vi "TrajectoryExecuteAbsolute.vi"(8 "Init":bool, 11 "End Pose ENG":T1={"TRANSLATION"={"X"=0.0, "Y"=0.0}, "ROTATION"={"VALUE"=0.0, "COS"=1.0, "SIN"=0.0}} {"ROTATION"."SIN" format="%13.4f"; "ROTATION"."COS" format="%13.4f"; "ROTATION"."VALUE" format="%13.4f"; "TRANSLATION"."Y" format="%14.3f"; "TRANSLATION"."X" format="%14.3f"}) -> (0 "AtReference":bool, 3 "Chassis Velocity Target":T4 {"vOmega" format="%10.3f"; "vY" format="%10.3f"; "vX" format="%10.3f"})   [LabVIEW 2023]
uses:
  <vilib>/Rock Robotics/WPI/ThirdParty/JAS_Junk/TrajLib/TypeDef/CHASSIS_SPEEDS.ctl
  <vilib>/Rock Robotics/WPI/ThirdParty/JAS_Junk/TrajLib/TypeDef/POSE2D.ctl
  <vilib>/Rock Robotics/WPI/ThirdParty/JAS_Junk/TrajLib/TypeDef/TRANSLATION2D.ctl
  <vilib>/Rock Robotics/WPI/ThirdParty/JAS_Junk/TrajLib/TypeDef/ROTATION2D.ctl
  <vilib>/Rock Robotics/WPI/ThirdParty/JAS_Junk/TrajLib/VI/Util_GetTime_U32.vi
  <vilib>/Rock Robotics/WPI/ThirdParty/JAS_Junk/TrajLib/HolDrvCtrl_New.vi
  <vilib>/Rock Robotics/WPI/ThirdParty/JAS_Junk/TrajLib/HolDrvCtrl_PackPID.vi
  <vilib>/Rock Robotics/WPI/ThirdParty/JAS_Junk/TrajLib/HolDrvCtrl_SetTolerance.vi
  <vilib>/Rock Robotics/WPI/ThirdParty/JAS_Junk/TrajLib/HolDrvCtrl_SetEnabled.vi
  <vilib>/Rock Robotics/WPI/ThirdParty/JAS_Junk/TrajLib/HolDrvCtrl_Calculate_Trajectory.vi
  <vilib>/Rock Robotics/WPI/ThirdParty/JAS_Junk/TrajLib/HolDrvCtrl_AtReference.vi
  <vilib>/Rock Robotics/WPI/ThirdParty/JAS_Junk/TrajLib/ProfiledPIDController_NewPeriod.vi
  <vilib>/Rock Robotics/WPI/ThirdParty/JAS_Junk/TrajLib/ProfiledPIDController_SetIntegratorRange.vi
  <vilib>/Rock Robotics/WPI/ThirdParty/JAS_Junk/TrajLib/ProfiledPIDController_DisableContInput.vi
  <vilib>/Rock Robotics/WPI/ThirdParty/JAS_Junk/TrajLib/ProfiledPIDController_EnableContInput.vi
  <vilib>/Rock Robotics/WPI/ThirdParty/JAS_Junk/TrajLib/TrapProfConstraint_New.vi
  <vilib>/Rock Robotics/WPI/ThirdParty/JAS_Junk/TrajLib/Rotation2d_CreateAngle.vi
  <vilib>/Rock Robotics/WPI/ThirdParty/JAS_Junk/TrajLib/Translation2d_Create.vi
  <vilib>/Rock Robotics/WPI/ThirdParty/JAS_Junk/TrajLib/Conv_Deg_Radians.vi
  <vilib>/Rock Robotics/WPI/ThirdParty/JAS_Junk/TrajLib/PIDController_NewPeriod.vi
  <vilib>/Rock Robotics/WPI/ThirdParty/JAS_Junk/TrajLib/PIDController_SetIntegratorRange.vi
  <vilib>/Rock Robotics/WPI/ThirdParty/JAS_Junk/TrajLib/PIDController_Reset.vi
  <vilib>/Rock Robotics/WPI/ThirdParty/JAS_Junk/TrajLib/HolDrvCtrl_Calculate.vi
  <vilib>/Rock Robotics/WPI/ThirdParty/JAS_Junk/TrajLib/Rotation2d_GetRadians.vi
  <vilib>/Rock Robotics/WPI/ThirdParty/JAS_Junk/TrajLib/TrapProfState_New.vi
  <vilib>/Rock Robotics/SystemInterfaces/NetworkCommunication/NetComm_UsageReport_report.vi
  <vilib>/Rock Robotics/WPI/ThirdParty/JAS_Junk/TrajLib/PIDController_DisableContinousInput.vi
  <vilib>/Rock Robotics/WPI/ThirdParty/JAS_Junk/TrajLib/PIDController_EnableContinousInput.vi
  <vilib>/Rock Robotics/WPI/ThirdParty/JAS_Junk/TrajLib/Rotation2d_GetAngleCosSin.vi
  <vilib>/Rock Robotics/WPI/ThirdParty/JAS_Junk/TrajLib/Pose2d_RelativeTo.vi
  <vilib>/Rock Robotics/WPI/ThirdParty/JAS_Junk/TrajLib/Pose2d_getRotation.vi
  <vilib>/Rock Robotics/WPI/ThirdParty/JAS_Junk/TrajLib/Rotation2d_Minus.vi
  <vilib>/Rock Robotics/WPI/ThirdParty/JAS_Junk/TrajLib/ProfiledPIDController_Calculate_Meas_Goal.vi
  <vilib>/Rock Robotics/WPI/ThirdParty/JAS_Junk/TrajLib/PIDController_Calculate_SP_PV.vi
  <vilib>/Rock Robotics/WPI/ThirdParty/JAS_Junk/TrajLib/ProfiledPIDController_Reset_PosOnly.vi
  <vilib>/Rock Robotics/WPI/ThirdParty/JAS_Junk/TrajLib/ChassisSpeeds_FromFieldRelativeSpeeds.vi
  <vilib>/Rock Robotics/WPI/ThirdParty/JAS_Junk/TrajLib/Transform2d_Create_PosePose.vi
  <vilib>/Rock Robotics/WPI/ThirdParty/JAS_Junk/TrajLib/Pose2d_New_TRRO.vi
  <vilib>/Rock Robotics/WPI/ThirdParty/JAS_Junk/TrajLib/Rotation2d_UnaryMinus.vi
  <vilib>/Rock Robotics/WPI/ThirdParty/JAS_Junk/TrajLib/Rotation2d_RotateBy.vi
  <vilib>/Rock Robotics/WPI/ThirdParty/JAS_Junk/TrajLib/ProfiledPIDController_SetGoal_PosOnly.vi
  <vilib>/Rock Robotics/WPI/ThirdParty/JAS_Junk/TrajLib/ProfiledPIDController_Calculate_Meas.vi
  <vilib>/Rock Robotics/WPI/ThirdParty/JAS_Junk/TrajLib/PIDController_SetSetpoint.vi
  <vilib>/Rock Robotics/WPI/ThirdParty/JAS_Junk/TrajLib/PIDController_Calculate_PV.vi
  <vilib>/Rock Robotics/WPI/ThirdParty/JAS_Junk/TrajLib/ProfiledPIDController_Reset.vi
  <vilib>/Rock Robotics/WPI/ThirdParty/JAS_Junk/TrajLib/Rotation2d_GetCos.vi
  <vilib>/Rock Robotics/WPI/ThirdParty/JAS_Junk/TrajLib/Rotation2d_GetSin.vi
  <vilib>/Rock Robotics/WPI/ThirdParty/JAS_Junk/TrajLib/Translation2d_RotateBy.vi
  <vilib>/Rock Robotics/WPI/ThirdParty/JAS_Junk/TrajLib/Translation2d_Minus.vi
  <vilib>/Rock Robotics/WPI/ThirdParty/JAS_Junk/TrajLib/Rotation2d_CreateXY.vi
  <vilib>/Rock Robotics/WPI/ThirdParty/JAS_Junk/TrajLib/ProfiledPIDController_SetGoal.vi
  <vilib>/Rock Robotics/WPI/ThirdParty/JAS_Junk/TrajLib/TrapProfile_New.vi
  <vilib>/Rock Robotics/WPI/ThirdParty/JAS_Junk/TrajLib/ProfiledPIDController_GetPeriod.vi
  <vilib>/Rock Robotics/WPI/ThirdParty/JAS_Junk/TrajLib/TrapProfile_Calculate.vi
  <vilib>/Rock Robotics/WPI/ThirdParty/JAS_Junk/TrajLib/ControllerUtil_GetModulusError.vi
  <vilib>/Rock Robotics/WPI/ThirdParty/JAS_Junk/TrajLib/Util_CalcDist.vi
  <vilib>/Rock Robotics/WPI/ThirdParty/JAS_Junk/TrajLib/TrapProfile_ShouldFlipAcceleration.vi
  <vilib>/Rock Robotics/WPI/ThirdParty/JAS_Junk/TrajLib/TrapProfile_Direct.vi
  <vilib>/Rock Robotics/WPI/ThirdParty/JAS_Junk/TrajLib/PIDController_GetPeriod.vi
  Vision/VisionGlobal.vi
  TrajectoryGlobals.vi
  <vilib>/Rock Robotics/SystemInterfaces/Utilities/FPGA_UtilitiesRead LocalTime.vi
  <vilib>/Rock Robotics/WPI/ThirdParty/JAS_Junk/TrajLib/VI/Util_GetTime_U64.vi
  <vilib>/Rock Robotics/WPI/ThirdParty/JAS_Junk/TrajLib/Globals/Util_LibraryGlobals.vi
  <vilib>/Rock Robotics/WPI/ThirdParty/JAS_Junk/TrajLib/Trajectory_Library.lvlib
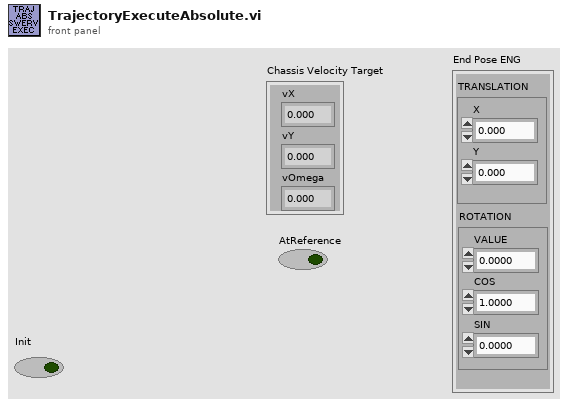
[diagram p1: front panel]
types:
  T1 = typedef "Trajectory_Library.lvlib/POSE2D.ctl" = cluster{"TRANSLATION":T2, "ROTATION":T3}
  T2 = typedef "Trajectory_Library.lvlib/TRANSLATION2D.ctl" = cluster{"X":dbl, "Y":dbl}
  T3 = typedef "Trajectory_Library.lvlib/ROTATION2D.ctl" = cluster{"VALUE":dbl, "COS":dbl, "SIN":dbl}
  T4 = typedef "Trajectory_Library.lvlib/CHASSIS_SPEEDS.ctl" = cluster{"vX":dbl, "vY":dbl, "vOmega":dbl}
  T5 = typedef "Trajectory_Library.lvlib/SWERVE_DRIVE_KINEMATICS.ctl" = cluster{"NumModules":i32, "InverseKinematics":T6, "ForwardKinematics":T6, "Modules":T2[], "PrevCoR":T2, "SavedModuleStates":T7[]}
  T6 = typedef "NI_Matrix.lvlib/RealMatrix.ctl" = dbl[][]
  T7 = typedef "Trajectory_Library.lvlib/SWERVE_DRIVE_MODULE_STATE.ctl" = cluster{"Speed":dbl, "Angle":T3}
  T8 = typedef "Trajectory_Library.lvlib/TRAJECTORY.ctl" = cluster{"TotalTImeSecs":dbl, "States":T9[]}
  T9 = typedef "Trajectory_Library.lvlib/TRAJ_STATE.ctl" = cluster{"TimeSeconds":dbl, "Velocity":dbl, "Acceleration":dbl, "POSE":T1, "Curvature":dbl}
  T10 = typedef "Trajectory_Library.lvlib/PID_TUNING.ctl" = cluster{"Kp":dbl, "Ki":dbl, "Kd":dbl, "MaximumIntegral":dbl, "MinimumIntegral":dbl, "IntegralZone":dbl}
  T11 = typedef "Trajectory_Library.lvlib/PROFILED_PID_CONTROLLER.ctl" = cluster{"Controller":T12, "Goal":T13, "Setpoint":T13, "Constraint":T14}
  T12 = typedef "Trajectory_Library.lvlib/PID_CONTROLLER.ctl" = cluster{"Kp":dbl, "Ki":dbl, "Kd":dbl, "Period":dbl, "Max_Integral":dbl, "Min_Integral":dbl, "Max_Input":dbl, "Min_Input":dbl, "Continuous":bool, "PositionError":dbl, "VelocityError":dbl, "PrevError":dbl, "Total_Integral":dbl, "PositionTolerance":dbl, "VelocityTolerance":dbl, "SetPoint":dbl, "Kf":dbl, "Prev_Deriv":dbl, "Prev_Deriv 2":dbl, "DerivativeFilter":bool, "Min_Output":dbl, "Max_Output":dbl, "Prev_F_P":dbl, "Prev_F_P_2":dbl, "AntiWindupActive":bool, "Measurement":dbl, "IntegralZone":dbl}
  T13 = typedef "Trajectory_Library.lvlib/TRAPEZOID_PROFILE_STATE.ctl" = cluster{"Position":dbl, "Velocity":dbl}
  T14 = typedef "Trajectory_Library.lvlib/TRAPEZOID_PROFILE_CONSTRAINT.ctl" = cluster{"MaxVelocity":dbl, "MaxAcceleration":dbl}
  T15 = typedef "Trajectory_Library.lvlib/HOLONOMIC_PACK_TUNING.ctl" = cluster{"X PID Tuning":T10, "Y PID Tuning":T10, "thetaProfiledPID_CTRL":T11}
  T16 = typedef "Trajectory_Library.lvlib/HOLONOMIC_DRV_CTRL.ctl" = cluster{"poseTolerance":T1, "poseError":T1, "Enabled":bool, "PID_xCtrl":T12, "PID_yCtrl":T12, "PROF_PID_thetaCtrl":T11, "RotationError":T3, "FirstRun":bool}
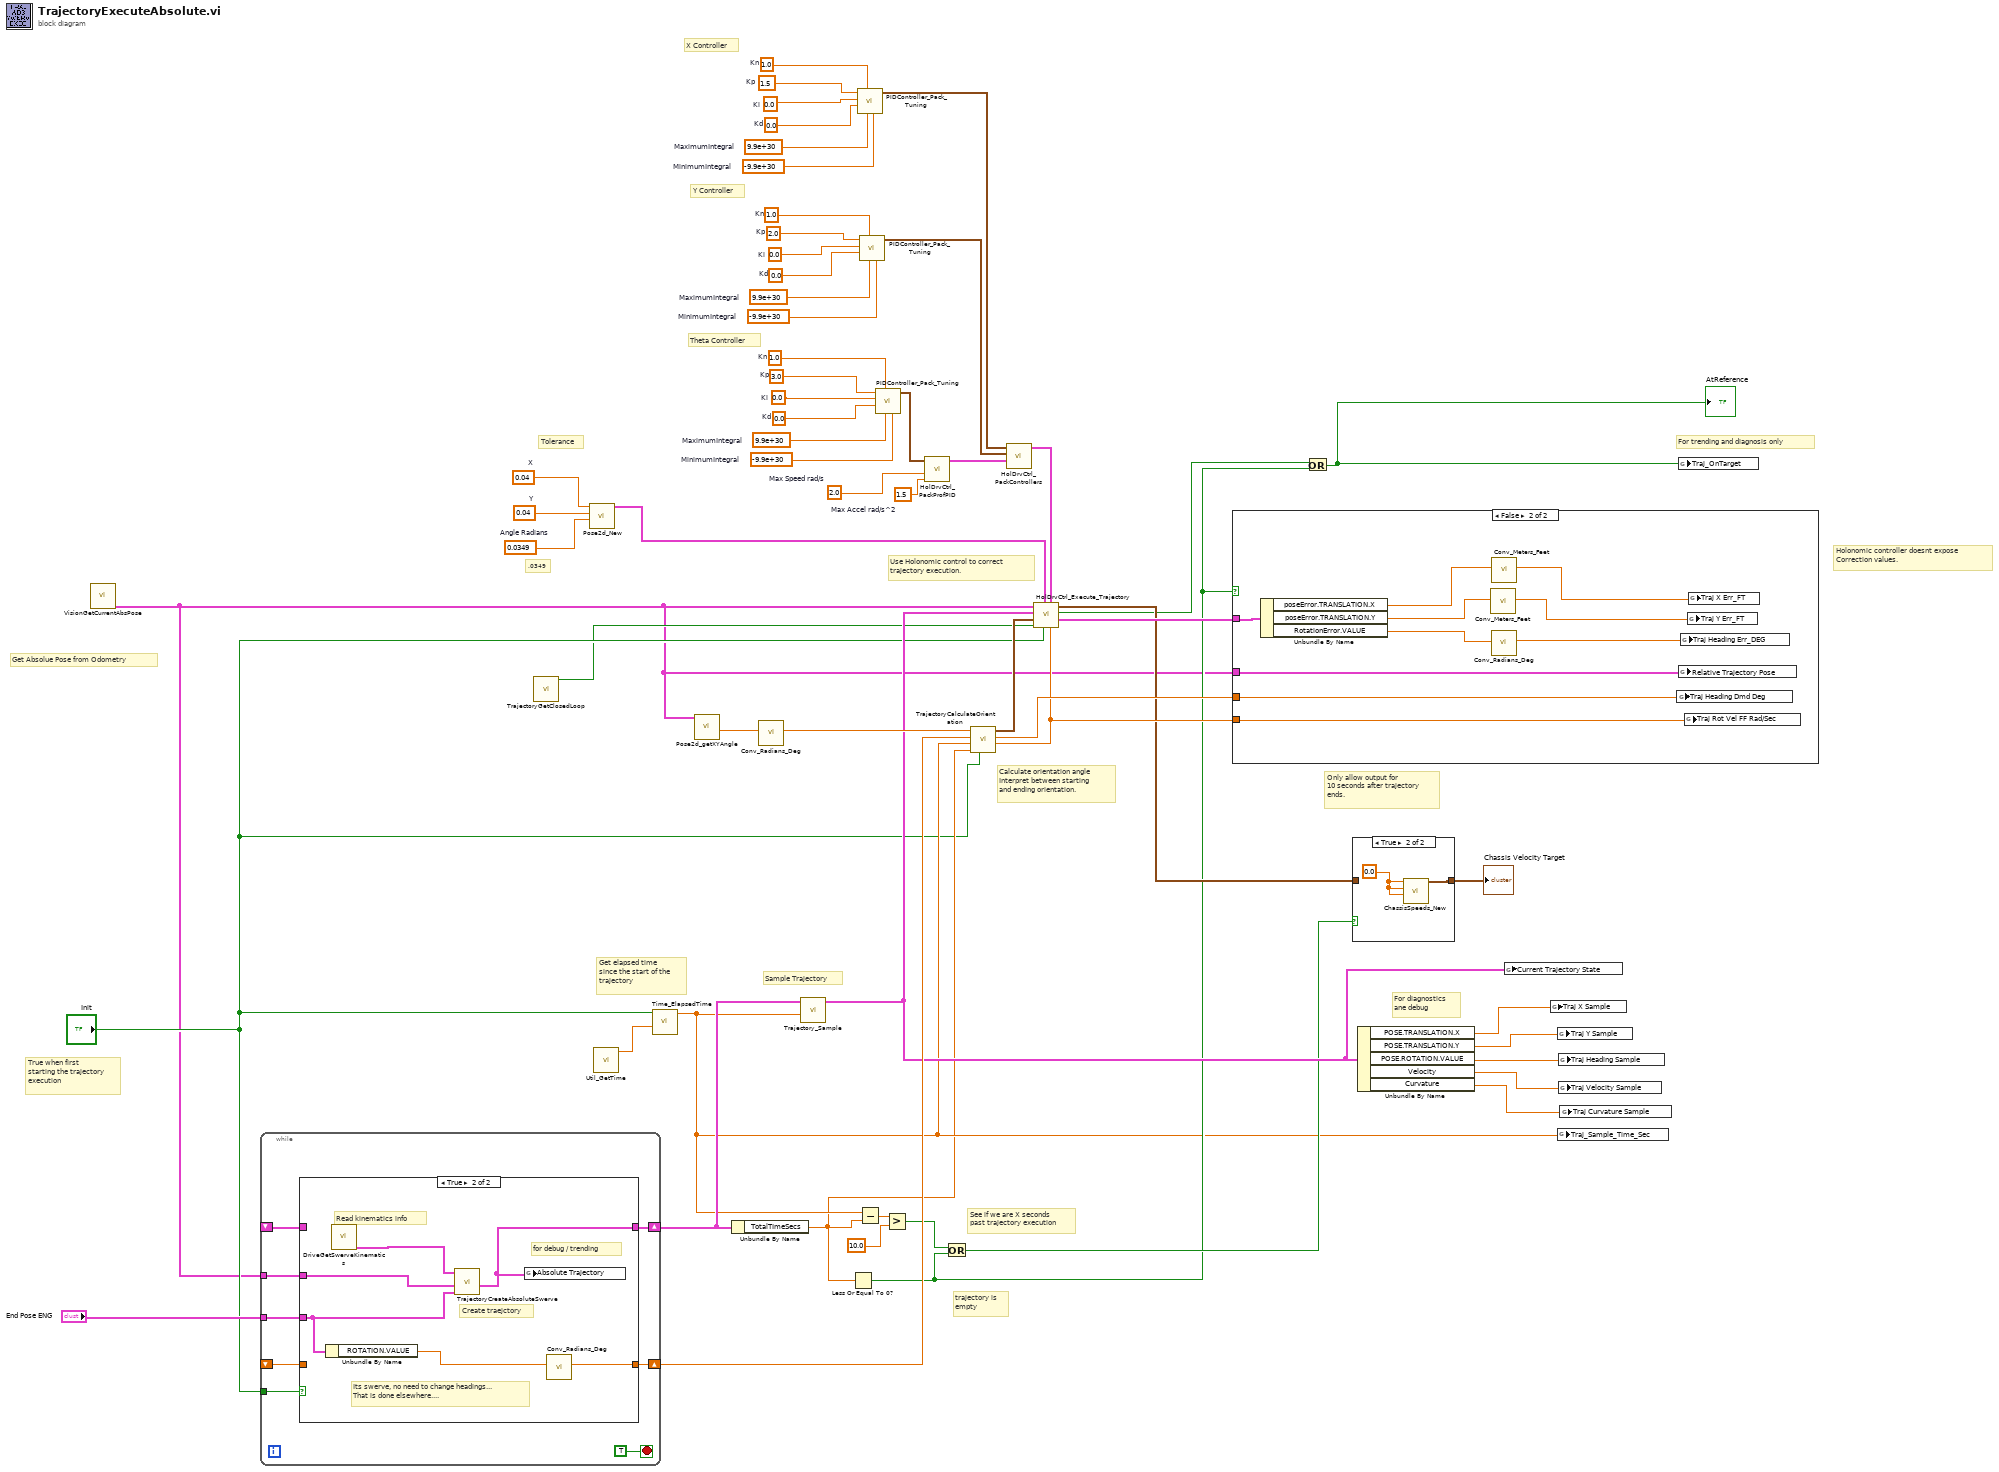
[diagram p0: block diagram]
diagram:
  w3 = 0.04  # X
  w2 = 0.04  # Y
  w4 = 0.0349  # Angle Radians
  w5 = 1.5  # Max Accel rad/s^2
  w6 = 2.0  # Max Speed rad/s
  w30 = 1.0  # Kn
  w33 = 3.0  # Kp
  w42 = 0.0  # Ki
  w43 = 0.0  # Kd
  w44 = 9.9e+30  # MaximumIntegral
  w45 = -9.9e+30  # MinimumIntegral
  w28 = 1.0  # Kn
  w31 = 1.5  # Kp
  w34 = 0.0  # Ki
  w35 = 0.0  # Kd
  w36 = 9.9e+30  # MaximumIntegral
  w37 = -9.9e+30  # MinimumIntegral
  w29 = 1.0  # Kn
  w32 = 2.0  # Kp
  w38 = 0.0  # Ki
  w39 = 0.0  # Kd
  w40 = 9.9e+30  # MaximumIntegral
  w41 = -9.9e+30  # MinimumIntegral
  # ".0349"
  # "Tolerance"
  # "trajectory is \nempty"
  # "Theta Controller"
  # "Y Controller"
  # "X Controller"
  # "Calculate orientation angle\nInterpret between starting\nand ending orientation."
  # "True when first\nstarting the trajectory\nexecution"
  # "Get elapsed time\nsince the start of the\ntrajectory"
  # "Holonomic controller doesnt expose\nCorrection values."
  # "Use Holonomic control to correct\ntrajectory execution."
  # "For trending and diagnosis only"
  # "For diagnostics\nane debug"
  # "Get Absolue Pose from Odometry"
  # "Sample Trajectory"
  # "See if we are X seconds \npast trajectory execution"
  # "Only allow output for\n10 seconds after trajectory\nends."
  n1 = call "VisionGetCurrentAbsPose.vi"() -> ("Current ABS Pose"=w7:T1)  [unwired: 9 in]
  n2 = while {
    tunnel: "Init" -> [w66]
    tunnel: w7 -> [w65]
    shift-right: [w64] -> w23
    shift-left: _ -> [w63]
    shift-right: [w62] -> w20
    shift-left: _ -> [w61]
    tunnel: "End Pose ENG" -> [w60]
    stop <- TRUE stop-if-true
    n3 = case shown="True" w66 {
      tunnel: w65 -> [_ w71]
      tunnel: [w69 w72] -> w64
      tunnel: w63 -> [w69 _]
      tunnel: [w68 w74] -> w62
      tunnel: w61 -> [w68 _]
      tunnel: w60 -> [_ w75]
      frame False {
      }
      frame True {
        # "for debug / trending"
        # "Read kinematics info"
        # "Its swerve, no need to change headings...\nThat is done elsewhere...."
        # "Create traejctory"
        n4 = Unbundle By Name(w75) -> ("ROTATION.VALUE"=w73:dbl)
        n5 = call "DriveGetSwerveKinematics.vi"() -> ("SWERVE_DRIVE_KINEMATICS"=w70:T5)  [unwired: 11 in]
        n6 = call "TrajectoryCreateAbsoluteSwerve.vi"("End Pose  ENG"=w75, "Current Pose SI"=w71, "SWERVE_DRIVE_KINEMATICS"=w70) -> ("Absolute Trajectory"=w72:T8)  [unwired: 6 in, 2 out]
        n7 = global write "TrajectoryGlobals.vi" "Absolute Trajectory"(w72) -> ()
        n8 = call <vilib>:"Conv_Radians_Deg.vi"("Radians"=w73) -> ("Degrees"=w74:dbl)  [unwired: 10 in]
      }
    }
  }
  n9 = call "TrajectoryGetClosedLoop.vi"() -> ("AUTO_CLOSED_LOOP"=w8:bool)  [unwired: 11 in]
  n10 = call <vilib>:"Pose2d_New.vi"("Heading"=w4, "Y"=w2, "X"=w3) -> ("out POSe"=w1:T1)  [unwired: 8 in]
  n11 = call <vilib>:"Util_GetTime.vi"() -> ("FPGA_Time_Seconds"=w56:dbl)  [unwired: 9 in, 2 out]
  n12 = call <vilib>:"Time_ElapsedTime.vi"("PassthroughTime_SEC"=w56, "Reset"="Init") -> ("Elapsed Time Sec"=w11:dbl)  [unwired: 9 in]
  n13 = call <vilib>:"Pose2d_getXYAngle.vi"("in POSE"=w7) -> ("Angle"=w22:dbl)  [unwired: 8 in, 2 out]
  n14 = Unbundle By Name(w23) -> ("TotalTImeSecs"=w10:dbl)
  n15 = call <vilib>:"Conv_Radians_Deg.vi"("Radians"=w22) -> ("Degrees"=w21:dbl)  [unwired: 10 in]
  n16 = call <vilib>:"Trajectory_Sample.vi"("Time"=w11, "InputTRAJECTORY"=w23) -> ("OutputTRAJ_STATE"=w19:T9)  [unwired: 9 in]
  n17 = Less Or Equal To 0?(x=w10) -> (x <= 0?=w12:bool)
  n18 = call <vilib>:"PIDController_Pack_Tuning.vi"("MinimumIntegral"=w37, "MaximumIntegral"=w36, "Kn"=w28, "Kd"=w35, "Ki"=w34, "Kp"=w31) -> ("PID Tuning"=w46:T10)  [unwired: 5 in]
  n19 = Subtract(x=w11, y=w10) -> (x-y=w59:dbl)
  n20 = call <vilib>:"PIDController_Pack_Tuning.vi"("MinimumIntegral"=w41, "MaximumIntegral"=w40, "Kn"=w29, "Kd"=w39, "Ki"=w38, "Kp"=w32) -> ("PID Tuning"=w47:T10)  [unwired: 5 in]
  n21 = call <vilib>:"PIDController_Pack_Tuning.vi"("MinimumIntegral"=w45, "MaximumIntegral"=w44, "Kn"=w30, "Kd"=w43, "Ki"=w42, "Kp"=w33) -> ("PID Tuning"=w27:T10)  [unwired: 5 in]
  n22 = Greater?(x=w59, y=10.0) -> (0:w16:bool)
  n23 = call <vilib>:"HolDrvCtrl_PackProfPID.vi"("Max Accel"=w5, "Max Speed"=w6, "Theta PID Tuning"=w27) -> ("Theta PID CONTROLLER"=w48:T11)  [unwired: 8 in]
  n24 = Or(x=w16, y=w12) -> (x .or. y?=w15:bool)
  n25 = call "TrajectoryCalculateOrientation.vi"("Init"="Init", "Total Trajectory Time Sec"=w10, "Elapsed Traj Time Sec"=w11, "End Orientation Demand DEG"=w20, "Starting Orientation  DEG"=w21) -> ("Rotational Velocity Rad Per Sec"=w24:dbl, "Orientation Demand Deg"=w50:dbl, "Orientation Demand"=w26:T3)  [unwired: 4 in]
  n26 = call <vilib>:"HolDrvCtrl_PackControllers.vi"("thetaProfiledPID_CTRL"=w48, "Y PID Tuning"=w47, "X PID Tuning"=w46) -> ("HOLONOMIC_CTRL_PACK_TUNING"=w49:T15)  [unwired: 8 in]
  n27 = call <vilib>:"HolDrvCtrl_Execute_Trajectory.vi"("Rotational Velocity Feedforward \nRad/Sec"=w24, "HOLONOMIC_CTRL_PACK_TUNING"=w49, "Reset"="Init", "Tolerance"=w1, "Enable"=w8, "angleRef"=w26, "desiredTrajState"=w19, "currentPose"=w7) -> ("outHOLONOMIC_DRV_CTRL"=w25:T16, "AtReference"=w14:bool, "calcChassisSpeed"=w17:T4)  [unwired: 1 in]
  n28 = case shown="False" w12 {
    tunnel: w50 -> [_ w85]
    tunnel: w25 -> [_ w79]
    tunnel: w24 -> [_ w78]
    tunnel: w7 -> [_ w76]
    frame True {
    }
    frame False {
      n29 = Unbundle By Name(w79) -> ("poseError.TRANSLATION.X"=w83:dbl, "poseError.TRANSLATION.Y"=w82:dbl, "RotationError.VALUE"=w77:dbl)
      n30 = call <vilib>:"Conv_Meters_Feet.vi"("Meters"=w82) -> ("Feet"=w81:dbl)  [unwired: 10 in]
      n31 = call <vilib>:"Conv_Radians_Deg.vi"("Radians"=w77) -> ("Degrees"=w84:dbl)  [unwired: 10 in]
      n32 = call <vilib>:"Conv_Meters_Feet.vi"("Meters"=w83) -> ("Feet"=w80:dbl)  [unwired: 10 in]
      n33 = global write "TrajectoryGlobals.vi" "Traj Heading Dmd Deg"(w85) -> ()
      n34 = global write "TrajectoryGlobals.vi" "Relative Trajectory Pose"(w76) -> ()
      n35 = global write "TrajectoryGlobals.vi" "Traj Heading Err_DEG"(w84) -> ()
      n36 = global write "TrajectoryGlobals.vi" "Traj Rot Vel FF Rad/Sec"(w78) -> ()
      n37 = global write "TrajectoryGlobals.vi" "Traj Y Err_FT"(w81) -> ()
      n38 = global write "TrajectoryGlobals.vi" "Traj X Err_FT"(w80) -> ()
    }
  }
  n39 = Or(x=w14, y=w12) -> (x .or. y?=w13:bool)
  "AtReference" <- w13
  n40 = case shown="True" w15 {
    tunnel: w17 -> [w86 _]
    tunnel: [w86 w87] -> w57
    frame False {
    }
    frame True {
      w88 = 0.0 ("vX")
      n41 = call <vilib>:"ChassisSpeeds_New.vi"("vAngular"=w88, "vY"=w88, "vX"=w88) -> ("CHASSIS"=w87:T4)  [unwired: 8 in]
    }
  }
  "Chassis Velocity Target" <- w57
  n42 = Unbundle By Name(w19) -> ("POSE.TRANSLATION.X"=w55:dbl, "POSE.TRANSLATION.Y"=w54:dbl, "POSE.ROTATION.VALUE"=w53:dbl, "Velocity"=w52:dbl, "Curvature"=w51:dbl)
  n43 = global write "TrajectoryGlobals.vi" "Current Trajectory State"(w19) -> ()
  n44 = global write "TrajectoryGlobals.vi" "Traj X Sample"(w55) -> ()
  n45 = global write "TrajectoryGlobals.vi" "Traj Y Sample"(w54) -> ()
  n46 = global write "TrajectoryGlobals.vi" "Traj_Sample_Time_Sec"(w11) -> ()
  n47 = global write "TrajectoryGlobals.vi" "Traj Heading Sample"(w53) -> ()
  n48 = global write "TrajectoryGlobals.vi" "Traj Velocity Sample"(w52) -> ()
  n49 = global write "TrajectoryGlobals.vi" "Traj Curvature Sample"(w51) -> ()
  n50 = global write "TrajectoryGlobals.vi" "Traj_OnTarget"(w13) -> ()
